vi "Ball Handling Controller.vi"(8 "error in":errorcluster) -> ()   [LabVIEW 2019]
doc: "This VI executes continuously carrying out the current operation and responding to updates or new operations. It will often contain the timing or control code that is difficult to place directly in TeleOp. This VI generally opens all sensors and motors and isolates the rest of the robot code from knowing how the operations are carried out."
uses:
  <vilib>/Rock Robotics/WPI/Framework/Completion Status.ctl
  Ball Handling Setpoints.ctl
  Ball Handling Operations.ctl
  <vilib>/Rock Robotics/WPI/Solenoid/WPI_SolenoidChannel.ctl
  <vilib>/Rock Robotics/WPI/Solenoid/WPI_SolenoidValue.ctl
  <vilib>/Rock Robotics/WPI/Solenoid/WPI_SolenoidOpenSingle.vi
  <vilib>/Rock Robotics/WPI/Solenoid/WPI_SolenoidSetEnum.vi
panel:
  in  "Interactive Values":T1
  out "Current\nCmd":string
  in  "Buttons":cluster{"Execute Cmd":bool, "Abort Cmd":bool}
  out "Command Timing":cluster{"Start Time (ms)":u32, "Iterations":i32}
  out "Status":T3
  # "Tip: It may be helpful to observe inputs and sensor values.\nYou may also want to display tuning or debugging controls."
  # "Interactive Command: You may fill in the settings for a command\nand schedule it with the Execute button. You can observe and abort\nany command while fine tuning the code for the controller."
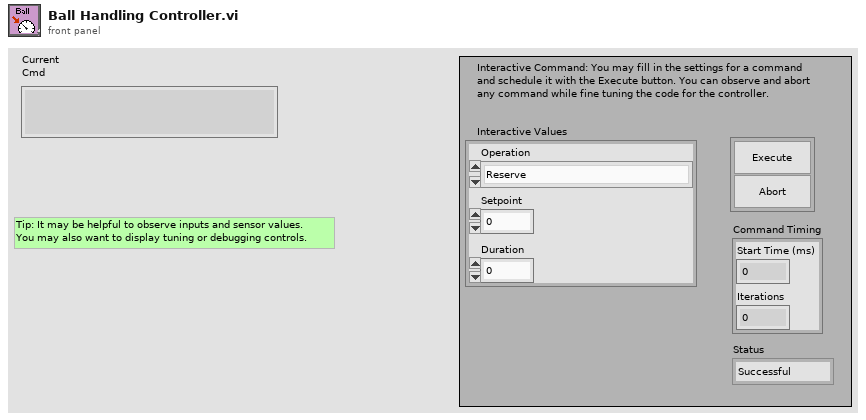
[diagram p1: front panel]
types:
  T1 = typedef "Ball Handling Setpoints.ctl" = cluster{"Operation":T2, "Setpoint":dbl, "Duration":dbl}
  T2 = typedef "Ball Handling Operations.ctl" = enum16{"Reserve", "Read Current", "Immediate", "Raise Intake", "Lower Intake", "Intake"}
  T3 = typedef "Completion Status.ctl" = enum16{"Successful", "Aborted", "Incomplete"}
  T4 = typedef "WPI_SolenoidChannel.ctl" = enum8{"Solenoid 0", "Solenoid 1", "Solenoid 2", "Solenoid 3", "Solenoid 4", "Solenoid 5", "Solenoid 6", "Solenoid 7", "Invalid"}
  T5 = typedef "WPI_SolenoidDevRef.ctl" = cluster{"DevStatus":errorcluster, "Pneumatics Control Module":u8, "Forward Solenoid Channel":T4, "Reverse Solenoid Channel":T4}
  T6 = typedef "WPI_CompressorDevRef.ctl" = cluster{"DevStatus":errorcluster, "Pneumatics Control Module":u8}
  T7 = typedef "WPI_MotorControlDeviceRef.ctl" = cluster{"DeviceStatus":errorcluster, "Type":T8, "PWM":cluster{"PWM Channel":T9, "DeadBand":T10}, "CAN":cluster{"Device Number":u8, "SetOutput VI Ref":variant, "GetOutput VI Ref":variant, "Enable VI Ref":variant, "Disable VI Ref":variant, "Data":variant}, "Invert":bool, "DIO PWM":cluster{"PWM \"Enable\" Channel":T9, "DIOChannel":T11, "PWM Rate":dbl}}
  T8 = typedef "WPI_MotorControlType.ctl" = enum16{"PWM", "CAN", "DIO PWM"}
  T9 = typedef "FPGA_DIOPWMChannel.ctl" = enum8{"PWM 0", "PWM 1", "PWM 2", "PWM 3", "PWM 4", "PWM 5", "PWM 6", "PWM 7", "PWM 8", "PWM 9", "PWM MXP 0", "PWM MXP 1", "PWM MXP 2", "PWM MXP 3", "PWM MXP 4", "PWM MXP 5", "PWM MXP 6", "PWM MXP 7", "PWM MXP 8", "PWM MXP 9", "Invalid"}
  T10 = typedef "WPI_PWMDeadband.ctl" = cluster{"Name":string, "maxPositivePwm":i32, "minPositivePwm":i32, "centerPwm":i32, "maxNegativePwm":i32, "minNegativePwm":i32, "angularRange":u16}
  T11 = typedef "FPGA_DIOChannel.ctl" = enum8{"DIO 0", "DIO 1", "DIO 2", "DIO 3", "DIO 4", "DIO 5", "DIO 6", "DIO 7", "DIO 8", "DIO 9", "DIO MXP 0", "DIO MXP 1", "DIO MXP 2", "DIO MXP 3", "DIO MXP 4", "DIO MXP 5", "DIO MXP 6", "DIO MXP 7", "DIO MXP 8", "DIO MXP 9", "DIO MXP 10", "DIO MXP 11", "DIO MXP 12", "DIO MXP 13", "DIO MXP 14", "DIO MXP 15", "SPI Port CS1", "SPI Port CS2", "SPI Port CS3", "SPI Port MISO", "SPI Port MOSI", "Invalid"}
  T12 = typedef "Command Status Info.ctl" = cluster{"Name":string, "Status":T3, "notifier out":T13}
  T13 = typedef "Completion Notifier.ctl" = refnum<notifier>
  T14 = cluster{"Current Command":T1, "Command Timing":cluster{"Start Time (ms)":u32, "Iterations":i32}, "Command Arguments":cluster{"Command Info":T12, "Description":string, "Default Command":T1, "queue out":refnum<queue>, "Subsystem Name":string}}
  T15 = typedef "WPI_SolenoidValue.ctl" = enum16{"Off", "On", "Forward", "Reverse"}
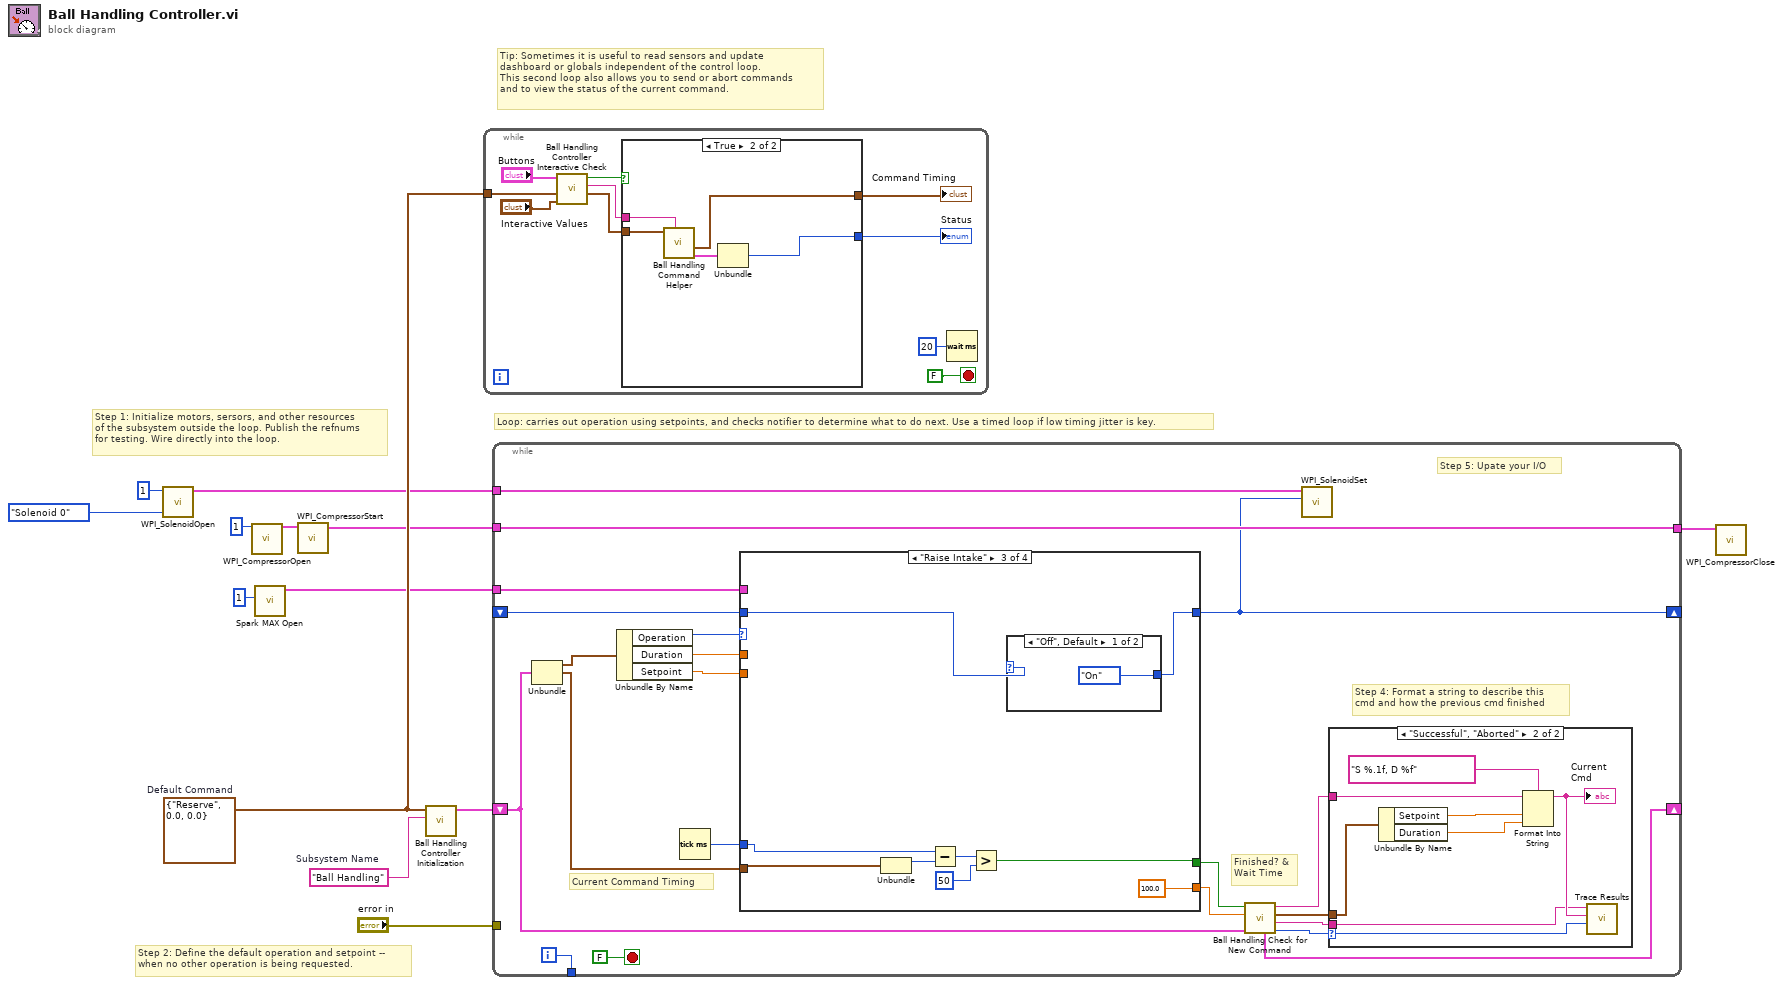
[diagram p0: block diagram]
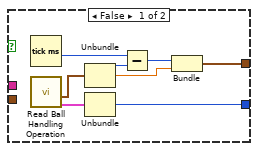
[diagram p2: hidden frame]
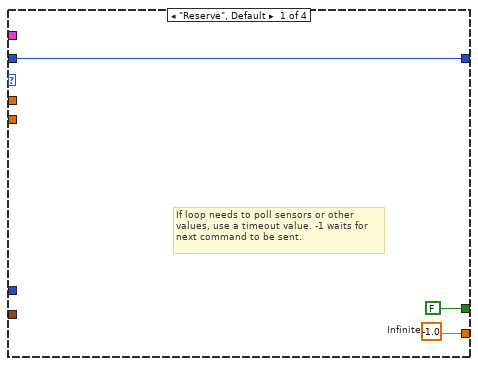
[diagram p4: hidden frame]
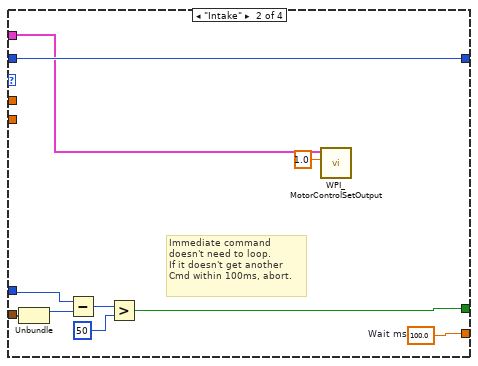
[diagram p5: hidden frame]
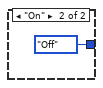
[diagram p6: hidden frame]
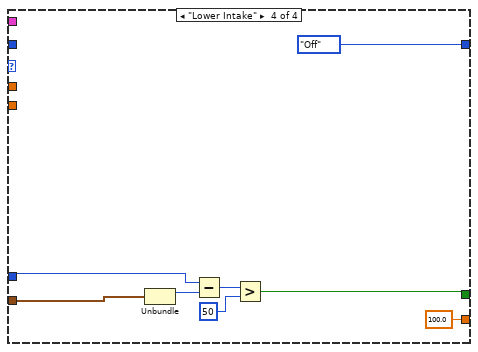
[diagram p7: hidden frame]
diagram:
  w10 = T1 {"Operation"=enum."Reserve", "Setpoint"=0.0, "Duration"=0.0}  # Default Command
  w11 = "Ball Handling"  # Subsystem Name
  # "Tip: Sometimes it is useful to read sensors and update\ndashboard or globals independent of the control loop.\nThis second loop also allows you to send or abort commands\nand to view the status of the current command."
  # "Step 2: Define the default operation and setpoint --\nwhen no other operation is being requested."
  # "Step 1: Initialize motors, sersors, and other resources\nof the subsystem outside the loop. Publish the refnums\nfor testing. Wire directly into the loop."
  # "Loop: carries out operation using setpoints, and checks notifier to determine what to do next. Use a timed loop if low timing jitter is key."
  n1 = call-poly <vilib>:"WPI_SolenoidOpen.vi"("Solenoid Channel"=WPI_SolenoidChannel."Solenoid 0", "Pneumatics Control Module (0)"=u8 1) -> ("SolenoidDevRef"=w5:T5)  [unwired: 8 in, 1 out]
  n2 = call <vilib>:"WPI_CompressorOpen.vi"("Pneumatics Control Module (0)"=u8 1) -> ("CompressorDevRef"=w3:T6)  [unwired: 13 in, 1 out]
  n3 = call <vilib>:"Spark MAX Open.vi"("Device Number"=u8 1) -> ("MotorControlDeviceRef"=w8:T7)  [unwired: 9 in, 1 out]
  n4 = call <vilib>:"WPI_CompressorStart.vi"("CompressorDevRef"=w3) -> ("CompressorDevRef"=w1:T6)  [unwired: 9 in, 1 out]
  n5 = call "Ball Handling Controller Initialization.vi"("Subsystem Name"=w11, "Default Command"=w10) -> ("Current Command"=w12:T14)  [unwired: 9 in]
  n6 = while {
    tunnel: w10 -> [w20]
    stop <- FALSE stop-if-true
    n7 = call "Ball Handling Controller Interactive Check.vi"("Interactive Command in"="Interactive Values", "Default Command"=w20, "Buttons"="Buttons") -> ("Interactive Command out"=w17:T1, "Trace String"=w18:string, "Schedule"=w19:bool)  [unwired: 6 in]
    n8 = case shown="True" w19 {
      tunnel: [w31 w36] -> w16
      tunnel: w17 -> [_ w34]
      tunnel: [w27 w32] -> w15
      tunnel: w18 -> [_ w35]
      frame False {
        n9 = Tick Count (ms)() -> (millisecond timer value=w26:u32)
        n10 = call "Read Ball Handling Operation.vi"() -> ("Command Info"=w24:T12, "SubSystem Data"=w25:T1)  [unwired: 9 in, 1 out]
        n11 = Unbundle(w25) -> ("Operation"=w30:T2, "Setpoint"=w28:dbl)  [unwired: 1 out]
        n12 = Unbundle(w24) -> ("Status"=w31:T3)  [unwired: 2 out]
        n13 = Subtract(x=w26, y=w30) -> (x-y=w29:u32)
        n14 = Bundle(w29, "Setpoint"=w28) -> (w27:cluster{u32, "Setpoint":dbl})  [unwired: 1 in]
      }
      frame True {
        n15 = call "Ball Handling Command Helper.vi"("Description"=w35, "SubSystem Data"=w34) -> ("Command Info Out"=w33:T12, "Command Timing"=w32:cluster{"Start Time (ms)":u32, "Iterations":i32})  [unwired: 7 in, 1 out]
        n16 = Unbundle(w33) -> ("Status"=w36:T3)  [unwired: 2 out]
      }
    }
    "Status" <- w16
    "Command Timing" <- w15
    n17 = Wait (ms)(milliseconds to wait=u32 20) -> ()  [unwired: 1 out]
  }
  n18 = while {
    shift-right: [w49] -> _
    shift-left: w12 -> [w42]
    tunnel: [w56] -> _
    tunnel: "error in" -> [_]
    tunnel: w8 -> [w41]
    shift-right: [w38] -> _
    shift-left: _ -> [w37]
    tunnel: w5 -> [w40]
    tunnel: [w39] -> w4
    tunnel: w1 -> [w39]
    i -> [w56]
    stop <- FALSE stop-if-true
    # "Step 5: Upate your I/O"
    # "Step 4: Format a string to describe this\ncmd and how the previous cmd finished"
    # "Current Command Timing"
    # "Finished? &\nWait Time"
    n19 = Unbundle(w42) -> ("Current Command"=w55:T1, "Command Timing"=w51:cluster{"Start Time (ms)":u32, "Iterations":i32})  [unwired: 1 out]
    n20 = Unbundle By Name(w55) -> ("Operation"=w54:T2, "Duration"=w53:dbl, "Setpoint"=w50:dbl)
    n21 = Tick Count (ms)() -> (millisecond timer value=w52:u32)
    n22 = case shown="\"Raise Intake\"" w54 {
      tunnel: [w68 w71 100.0 ("Wait ms") 100.0 ("Wait ms")] -> w47
      tunnel: [FALSE ("ignore previous (F)") w74 w84 w94] -> w48
      tunnel: w51 -> [_ w72 w81 w92]
      tunnel: w53 -> [_ _ _ _]
      tunnel: w52 -> [_ w73 w82 w91]
      tunnel: w50 -> [_ _ _ _]
      tunnel: w41 -> [_ w69 _ _]
      tunnel: [w66 w70 w79 WPI_SolenoidValue."Off" ("Value")] -> w38
      tunnel: w37 -> [w66 w70 w80 _]
      frame "Reserve", Default {
        w68 = -1.0  # Infinite
        # "If loop needs to poll sensors or other\nvalues, use a timeout value. -1 waits for\nnext command to be sent."
      }
      frame "Intake" {
        w71 = 100.0  # Wait ms
        # "Immediate command\ndoesn't need to loop.\nIf it doesn't get another\nCmd within 100ms, abort."
        n23 = Unbundle(w72) -> ("Start Time (ms)"=w77:u32)  [unwired: 1 out]
        n24 = Subtract(x=w73, y=w77) -> (x-y=w76:u32)
        n25 = Greater?(x=w76, y=u8 50 ("Left Motor")) -> (0:w74:bool)
        n26 = call <vilib>:"WPI_MotorControlSetOutput.vi"("Output"=1.0, "MotorControlDevRef"=w69) -> ()  [unwired: 7 in, 3 out]
      }
      frame "Raise Intake" {
        n27 = Unbundle(w81) -> ("Start Time (ms)"=w87:u32)  [unwired: 1 out]
        n28 = Subtract(x=w82, y=w87) -> (x-y=w86:u32)
        n29 = Greater?(x=w86, y=u8 50 ("Left Motor")) -> (0:w84:bool)
        n30 = case shown="\"Off\", Default" w80 {
          tunnel: [WPI_SolenoidValue."On" ("Value") WPI_SolenoidValue."Off" ("Value")] -> w79
          frame "Off", Default {
          }
          frame "On" {
          }
        }
      }
      frame "Lower Intake" {
        n31 = Unbundle(w92) -> ("Start Time (ms)"=w96:u32)  [unwired: 1 out]
        n32 = Subtract(x=w91, y=w96) -> (x-y=w97:u32)
        n33 = Greater?(x=w97, y=u8 50 ("Left Motor")) -> (0:w94:bool)
      }
    }
    n34 = call "Ball Handling Check for New Command.vi"("Current Command"=w42, "Wait time (ms)"=w47, "Finished?"=w48) -> ("Completion"=w43:T3, "Subsystem Name"=w44:string, "Current Command"=w45:T1, "Initial Trace String"=w46:string, "NextCommand"=w49:T14)  [unwired: 4 in]
    n35 = call-poly <vilib>:"WPI_SolenoidSet.vi"("Value"=w38, "SolenoidDevRef"=w40) -> ()  [unwired: 8 in, 2 out]
    n36 = case shown="\"Successful\", \"Aborted\"" w43 {
      selector: w43 -> [_ w65]
      tunnel: w46 -> [_ w61]
      tunnel: w45 -> [_ w62]
      tunnel: w44 -> [_ w58]
      frame "Incomplete", Default {
        # "Continuing current command"
      }
      frame "Successful", "Aborted" {
        # "Report and setup for next command"
        n37 = Unbundle By Name(w62) -> ("Setpoint"=w64:dbl, "Duration"=w59:dbl)
        n38 = Format Into String(format string="S %.1f, D %f", initial string=w61, w64, w59) -> (resulting string=w60:string)  [unwired: 1 in, 1 out]
        "Current\nCmd" <- w60
        n39 = call <vilib>:"Trace Results.vi"("Status of previous command"=w65, "Description"=w60, "Subsystem"=w58) -> ()  [unwired: 9 in]
      }
    }
  }
  n40 = call <vilib>:"WPI_CompressorClose.vi"("CompressorDevRef"=w4) -> ()  [unwired: 10 in, 1 out]
